vi "StoreInFile.vi"(0 "FileName":string="data", 1 "show patch":bool, 2 "delimiter":string="\t", 3 "String":string, 4 "format":string="%.3f") -> ()   [LabVIEW 2018]
uses:
  <vilib>/Utility/file.llb/Write Delimited Spreadsheet (string).vi
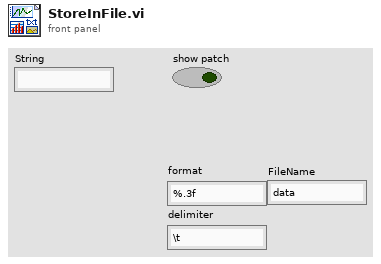
[diagram p1: front panel]
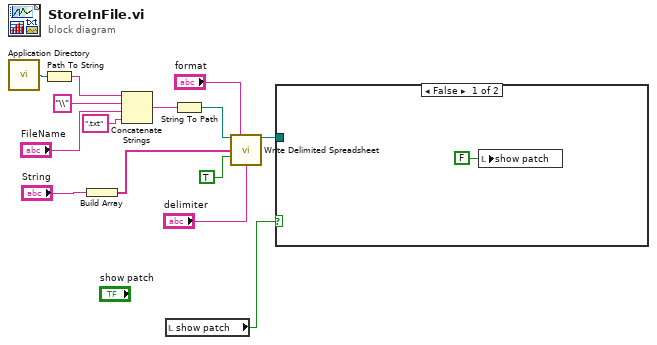
[diagram p0: block diagram]
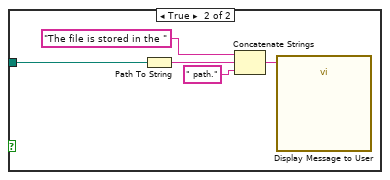
[diagram p2: hidden frame]
diagram:
  n1 = call <vilib>:"Application Directory.vi"() -> ("Application Directory"=w6:path)
  n2 = Path To String(path=w6) -> (string=w10:string)
  n3 = Build Array("String") -> (w3:string[])
  n4 = Concatenate Strings(w10, "\\" ("string"), "FileName", ".txt" ("string")) -> (w13:string)
  n5 = local read "show patch"() -> (w1:bool)
  n6 = String To Path(string=w13) -> (path=w11:path)
  n7 = call-poly <vilib>:"Write Delimited Spreadsheet.vi"("file path (dialog if empty)"=w11, "format (%s)"="format", "1D data"=w3, "append to file? (new file:F)"=TRUE, "delimiter (\\t)"="delimiter") -> ("new file path (Not A Path if cancelled)"=w9:path)  [unwired: 9 in, 1 out]
  n8 = case shown="False" w1 {
    tunnel: w9 -> [_ w20]
    frame False {
      n9 = local write "show patch"(FALSE ("show patch")) -> ()
    }
    frame True {
      n10 = Path To String(path=w20) -> (string=w18:string)
      n11 = Concatenate Strings("The file is stored in the " ("string"), w18, " path." ("string")) -> (w17:string)
      n12 = call "Display Message to User"("Message"=w17) -> ()  [unwired: 9 in, 2 out]
    }
  }
